vi "test simple.vi"() -> ()   [LabVIEW 2019, in "infolib.lvlib"]
uses:
  infolib.lvlib
  2D EXT.vi
  2D String.vi
  2D Time Stamp.vi
  GetI64.vi
  Get 2D EXT.vi
  Get 2D String.vi
  Get 2D Time Stamp.vi
panel:
  in  "time matrix":timestamp[][](array[timestamp])=[[timestamp(3541442244.3093777 s since 1904-01-01), timestamp(3541442247.373784 s since 1904-01-01)], [timestamp(3541443022.338128 s since 1904-01-01), timestamp(3541443027.89612 s since 1904-01-01)]]
  in  "time matrix key":string="string matrix"
  in  "string matrix key":string="string matrix"
  in  "string mat":string[][](array[string])=[["a", "b\nb"], ["c\"c", "d"]]
  in  "matrix":dbl[][](array[numeric])=[[1.0, 2.0], [3.0, 5.5]]
  in  "matrix key":string="somematrix"
  out "reading from\ninfo ok?":bool
  in  "value 2":i64=2
  in  "value after long insert":i64=5
  in  "key after long insert":string="key after long insert"
  in  "key 1":string="number test1 (A)"
  in  "key 2":string="number test2 $\\"
  in  "to insert":string="TEST string\nthat will be \ninserted\n!@#$%^&*()"
  in  "sections 2":string[](array[string])=["adc u calibration data"]
  out "joining two info strings:":string
  in  "sections":string[](array[string])=["section 1", "section 2"]
  in  "value 1":i64=1
  out "section do not exist, section is set":string
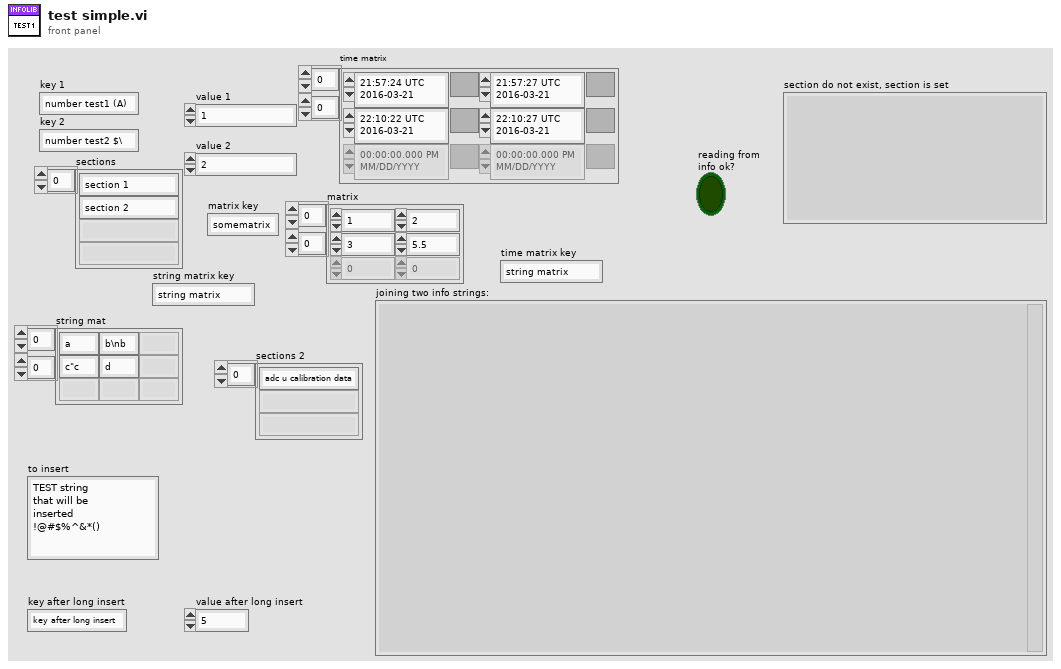
[diagram p1: front panel]
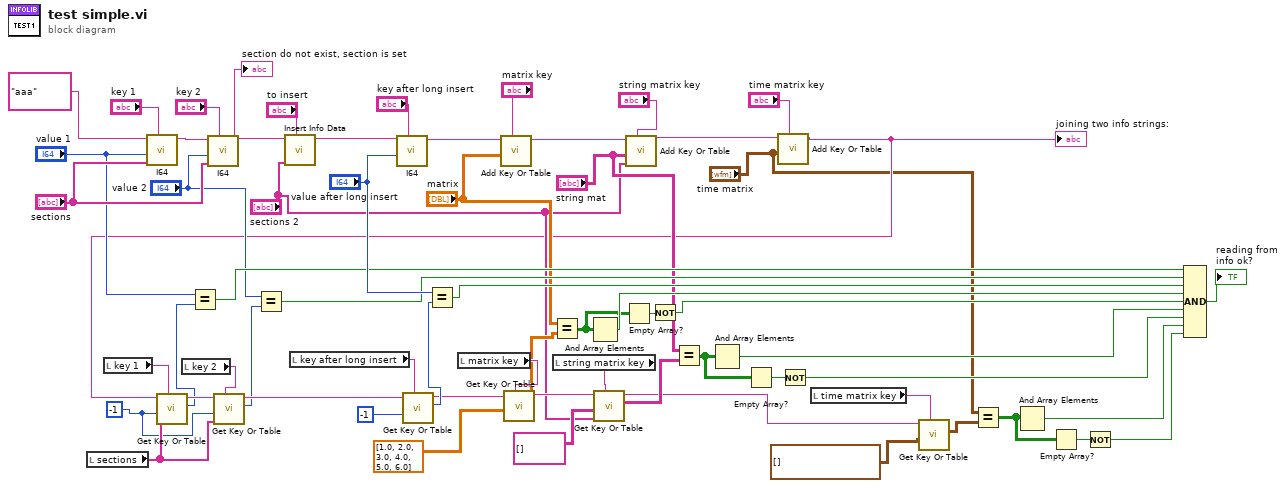
[diagram p0: block diagram]
diagram:
  w49 = i64 -1 ("values")
  n1 = local read "sections"() -> (w50:string[])
  n2 = local read "key 1"() -> (w53:string)
  n3 = call "I64.vi"("key description"="key 1", "sections"="sections", "numeric"="value 1", "info data"="aaa") -> ("info data out"=w60:string)  [unwired: 6 in, 1 out]
  n4 = local read "key 2"() -> (w51:string)
  n5 = call "I64.vi"("key description"="key 2", "sections"="sections", "numeric"="value 2", "info data"=w60) -> ("info data out"=w58:string)  [unwired: 6 in, 1 out]
  "section do not exist, section is set" <- w58
  n6 = call "Insert Info Data.vi"("info data to insert"="to insert", "sections"="sections 2", "info data"=w58) -> ("info data out"=w57:string)  [unwired: 7 in, 1 out]
  n7 = local read "key after long insert"() -> (w36:string)
  n8 = call "I64.vi"("key description"="key after long insert", "numeric"="value after long insert", "info data"=w57) -> ("info data out"=w35:string)  [unwired: 7 in, 1 out]
  n9 = local read "matrix key"() -> (w31:string)
  n10 = call-poly "Add Key Or Table.vi"("key description"="matrix key", "numeric"="matrix", "info data"=w35) -> ("info data out"=w27:string)  [unwired: 7 in, 1 out]
  n11 = local read "string matrix key"() -> (w25:string)
  n12 = call-poly "Add Key Or Table.vi"("key description"="string matrix key", "sections"="sections 2", "string"="string mat", "info data"=w27) -> ("info data out"=w12:string)  [unwired: 6 in, 1 out]
  n13 = call-poly "Add Key Or Table.vi"("key description"="time matrix key", "time stamp"="time matrix", "info data"=w12) -> ("info data out"=w11:string)  [unwired: 7 in, 1 out]
  "joining two info strings:" <- w11
  n14 = call-poly "Get Key Or Table.vi"("key description"=w53, "sections"=w50, "numeric"=w49, "info data"=w11) -> ("value"=w44:i64, "info data out"=w52:string)  [unwired: 5 in, 1 out]
  n15 = Equal?(x="value 1", y=w44) -> (x = y?=w41:bool)
  n16 = call-poly "Get Key Or Table.vi"("key description"=w51, "sections"=w50, "numeric"=w49, "info data"=w52) -> ("value"=w43:i64, "info data out"=w48:string)  [unwired: 5 in, 1 out]
  n17 = Equal?(x="value 2", y=w43) -> (x = y?=w40:bool)
  n18 = call-poly "Get Key Or Table.vi"("key description"=w36, "numeric"=i64 -1 ("values"), "info data"=w48) -> ("value"=w46:i64, "info data out"=w32:string)  [unwired: 6 in, 1 out]
  n19 = Equal?(x="value after long insert", y=w46) -> (x = y?=w39:bool)
  n20 = call-poly "Get Key Or Table.vi"("key description"=w31, "numeric"=dbl[][] [[1.0, 2.0], [3.0, 4.0], [5.0, 6.0]] ("matrix 2"), "info data"=w32) -> ("value"=w30:ext[][], "info data out"=w22:string)  [unwired: 6 in, 1 out]
  n21 = Equal?(x="matrix", y=w30) -> (x = y?=w16:bool[][])
  n22 = And Array Elements(Boolean array=w16) -> (logical AND=w28:bool)
  n23 = call-poly "Get Key Or Table.vi"("key description"=w25, "sections"="sections 2", "string"=string[][] [] ("string mat 2"), "info data"=w22) -> ("value"=w21:string[][], "info data out"=w8:string)  [unwired: 5 in, 1 out]
  n24 = Empty Array?(array=w16) -> (empty?=w17:bool)
  n25 = Not(x=w17) -> (.not. x?=w15:bool)
  n26 = Equal?(x="string mat", y=w21) -> (x = y?=w20:bool[][])
  n27 = And Array Elements(Boolean array=w20) -> (logical AND=w23:bool)
  n28 = Empty Array?(array=w20) -> (empty?=w19:bool)
  n29 = Not(x=w19) -> (.not. x?=w18:bool)
  n30 = local read "time matrix key"() -> (w9:string)
  n31 = call-poly "Get Key Or Table.vi"("key description"=w9, "time stamp"=timestamp[][] [] ("time matrix"), "info data"=w8) -> ("value"=w6:timestamp[][])  [unwired: 6 in, 2 out]
  n32 = Equal?(x="time matrix", y=w6) -> (x = y?=w3:bool[][])
  n33 = And Array Elements(Boolean array=w3) -> (logical AND=w2:bool)
  n34 = Empty Array?(array=w3) -> (empty?=w4:bool)
  n35 = Not(x=w4) -> (.not. x?=w1:bool)
  n36 = Compound Arithmetic op=AND(w41, w40, w39, w28, w15, w23, w18, w2, w1) -> (→"reading from\ninfo ok?":bool)
